vi "makeFitPlotCommands.vi"(5 "Fit Zmin":dbl=500.0 min=0.0, 6 "plotInfoArray":T1(array[cluster]), 7 "Fit Zmax":dbl=500.0 min=0.0, 9 "BL Targets":T2[](array[typedef]) {"n" min=0.02 max=0.5 step=0.01 format="%.2f"}, 10 "Coefficients":T3, 11 "Zref":dbl=508.0 min=0.0) -> (1 "UnderlayPlotSeries":string[](array[string])=["fitmin = 100, fitmax=550, zref=508, d=16.2, n=0.121, clippedpowerlaw(x) w line ls 1 lw 10 lc rgb \"gray25\" title 'fit with displacement'", "fitmin = 100, fitmax=550, zref=508, d=0, n=0.133, clippedpowerlaw(x) w line ls 1 lw 8 lc rgb \"gray50\" title 'zero displacement fit'", "zref=508, d=0, n=0.170, powerlaw(x) w line ls 0 lw 1 lc rgb \"gray75\" title 'target power law'"], 2 "Pre-plot Injection":string)   [LabVIEW 2013]
uses:
  BLTarget.ctl
  at.ctl
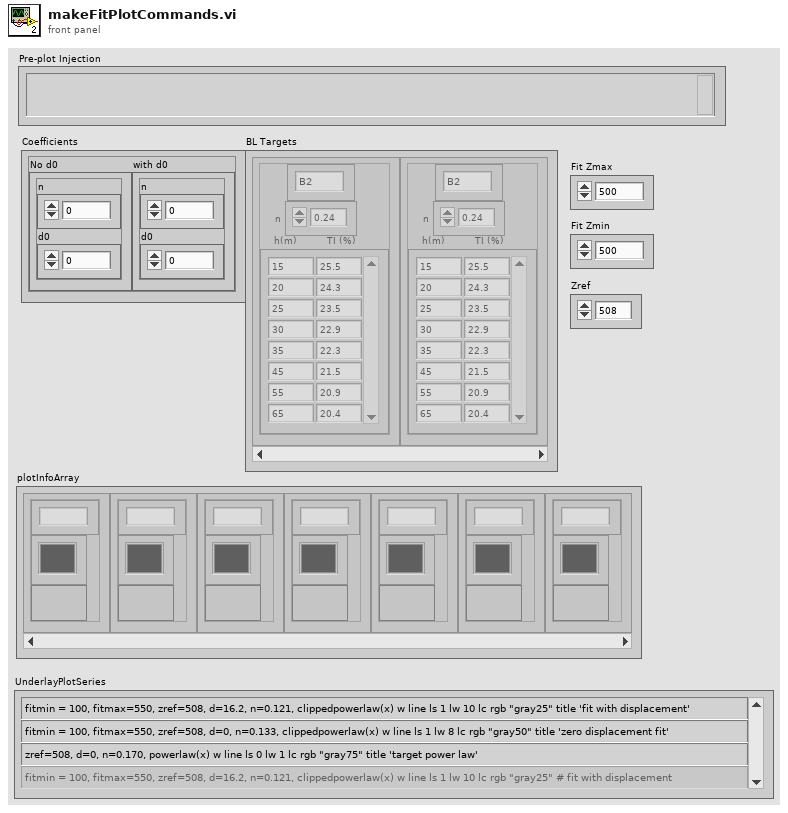
[diagram p1: front panel]
types:
  T1 = cluster{"Plot Name":string, "Plot.Plot Color":u32, "Plot.Visible?":bool}[]
  T2 = typedef "BLTarget.ctl" = cluster{"Code":string, "TI Profile (FS)":dbl[][], "n":dbl}
  T3 = cluster{"No d0":cluster{"n":dbl, "d0":dbl}, "with d0":cluster{"n":dbl, "d0":dbl}}
  T4 = typedef "at.ctl" = cluster{"XcoordSys":string, "YcoordSys":string, "Xvalue":dbl, "Yvalue":dbl}
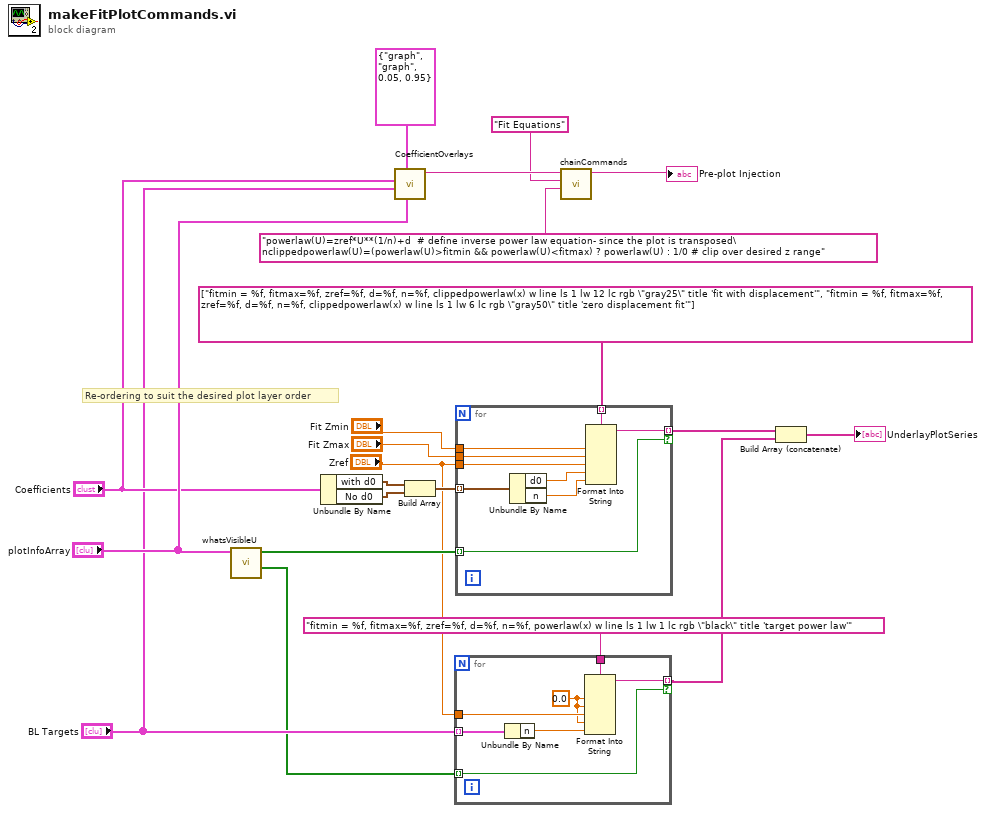
[diagram p0: block diagram]
diagram:
  # "Re-ordering to suit the desired plot layer order"
  n1 = call "whatsVisibleU.vi"("UplotInfoArray"="plotInfoArray") -> ("Targets Visible"=w1:bool[], "Fits Visible"=w11:bool[])  [unwired: 9 in]
  n2 = Unbundle By Name("Coefficients") -> ("with d0"=w20:cluster{"n":dbl, "d0":dbl}, "No d0"=w19:cluster{"n":dbl, "d0":dbl})
  n3 = call "CoefficientOverlays.vi"("plotInfoArray"="plotInfoArray", "\"At\" location"=T4 {"XcoordSys"="graph", "YcoordSys"="graph", "Xvalue"=0.05, "Yvalue"=0.95} ("\"At\" location"), "BL Targets"="BL Targets", "fitCoefficients"="Coefficients") -> ("gnuplotOut"=w15:string)  [unwired: 7 in]
  n4 = Build Array(w20, w19) -> (w17:cluster{"n":dbl, "d0":dbl}[])
  n5 = for {
    tunnel: "fitmin = %f, fitmax=%f, zref=%f, d=%f, n=%f, powerlaw(x) w line ls 1 lw 1 lc rgb \"black\" title 'target power law'" ("String") -> [w28]
    tunnel: "BL Targets" -> [w27] mode=indexing
    tunnel: [w26] -> w5 mode=indexing if=w22
    tunnel: w1 -> [w22] mode=indexing
    tunnel: "Zref" -> [w25]
    w24 = 0.0 ("input 1")
    n6 = Unbundle By Name(w27) -> ("n"=w23:dbl)
    n7 = Format Into String(format string=w28, w24, w24, w25, w24, w23) -> (resulting string=w26:string)  [unwired: 2 in, 1 out]
  }
  n8 = for {
    tunnel: string[] ["fitmin = %f, fitmax=%f, zref=%f, d=%f, n=%f, clippedpowerlaw(x) w line ls 1 lw 12 lc rgb \"gray25\" title 'fit with displacement'", "fitmin = %f, fitmax=%f, zref=%f, d=%f, n=%f, clippedpowerlaw(x) w line ls 1 lw 6 lc rgb \"gray50\" title 'zero displacement fit'"] ("UnderlayPlotSeries 2") -> [w37] mode=indexing
    tunnel: w17 -> [w36] mode=indexing
    tunnel: "Fit Zmin" -> [w35]
    tunnel: "Fit Zmax" -> [w34]
    tunnel: [w31] -> w16 mode=indexing if=w29
    tunnel: w11 -> [w29] mode=indexing
    tunnel: "Zref" -> [w30]
    n9 = Unbundle By Name(w36) -> ("d0"=w33:dbl, "n"=w32:dbl)
    n10 = Format Into String(format string=w37, w35, w34, w30, w33, w32) -> (resulting string=w31:string)  [unwired: 2 in, 1 out]
  }
  n11 = call "chainCommands.vi"("Command"="powerlaw(U)=zref*U**(1/n)+d  # define inverse power law equation- since the plot is transposed\nclippedpowerlaw(U)=(powerlaw(U)>fitmin && powerlaw(U)<fitmax) ? powerlaw(U) : 1/0 # clip over desired z range" ("FitEquations"), "Comments"="Fit Equations", "StringIn"=w15) -> ("StringOut"=→"Pre-plot Injection":string)  [unwired: 8 in]
  n12 = Build Array (concatenate)(w16, w5) -> (→"UnderlayPlotSeries":string[])
